vi "sine_wave.vi"(3 "output control":T1, 4 "data":variant, 5 "X":dbl[](array[numeric]), 6 "a":dbl[](array[numeric])) -> (0 "error out":errorcluster, 1 "f'(X,a)":dbl[][](array[numeric]), 2 "f(X,a)":dbl[](array[numeric]))   [LabVIEW 2011]
uses:
  <vilib>/gmath/NumericalOptimization/LM_output select.ctl
  <vilib>/gmath/NI_Gmath.lvlib
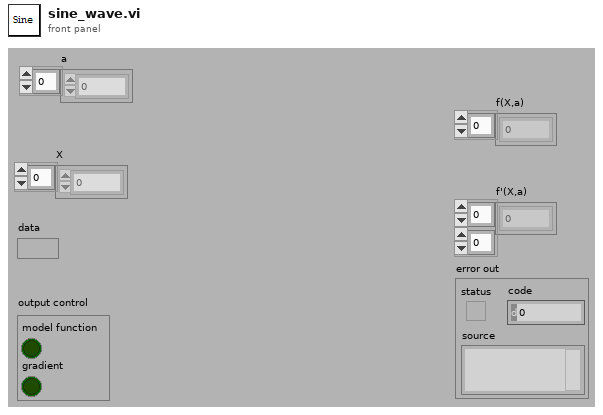
[diagram p1: front panel]
types:
  T1 = typedef "NI_Gmath.lvlib/LM_output select.ctl" = cluster{"model function":bool, "gradient":bool}
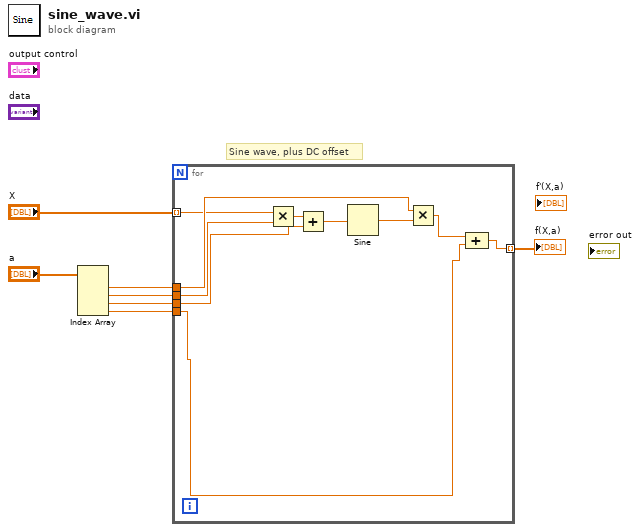
[diagram p0: block diagram]
diagram:
  # "Sine wave, plus DC offset"
  n1 = Index Array(array="a") -> (element #1=w6:dbl, element #2=w1:dbl, element #3=w5:dbl, element #4=w4:dbl)  [unwired: 4 in]
  n2 = for {
    tunnel: "X" -> [w13] mode=indexing
    tunnel: w6 -> [w17]
    tunnel: w1 -> [w12]
    tunnel: w5 -> [w10]
    tunnel: w4 -> [w8]
    tunnel: [w15] -> w3 mode=indexing
    n3 = Multiply(x=w13, y=w12) -> (x*y=w11:dbl)
    n4 = Add(x=w11, y=w10) -> (x+y=w9:dbl)
    n5 = Sine(x=w9) -> (sin(x)=w14:dbl)
    n6 = Multiply(x=w17, y=w14) -> (x*y=w16:dbl)
    n7 = Compound Arithmetic op=ADD(w16, w8) -> (w15:dbl)
  }
  "f(X,a)" <- w3
